vi "Lookup Manager.vi"(8 "error in (no error)":errorcluster, 11 "GUI Helper in":refnum<class "GUI Helper.lvclass">) -> (0 "error out":errorcluster, 3 "GUI Helper out":refnum<class "GUI Helper.lvclass">)   [LabVIEW 2020, in "VolatusGUI.lvlib" / "GUI Helper.lvclass"]
uses:
  GUI Helper.lvclass
  C:/dev/lv20CE/relink/lv-volatus/Volatus/Module/Module.lvclass
  Volatus/GUI Manager Identity/GUI Manager Identity.lvclass
  C:/dev/lv20CE/relink/lv-volatus/Volatus/Identity/Identity.lvclass
  Volatus/Module/Module.lvclass/Module.ctl
  GUI Helper.lvclass/GUI Helper.ctl
  GUI Registration.ctl
  Volatus/MessageQ/MessageQ.lvclass
  Volatus/MessageQ/MessageQ.lvclass/MessageQ.ctl
  Volatus/VolatusAPI/VolatusAPI.lvclass
  Volatus/Module/Module.lvclass
  VolatusGUI.lvlib
  GUI Info.ctl
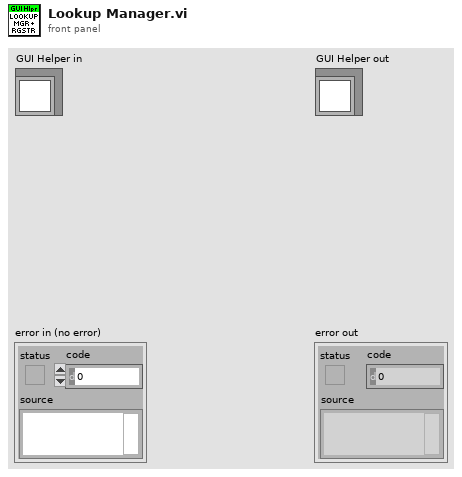
[diagram p1: front panel]
types:
  T1 = typedef "VolatusGUI.lvlib/GUI Info.ctl" = cluster{"Color":u32, "Name":string}
  T2 = typedef "VolatusGUI.lvlib/GUI Registration.ctl" = cluster{"ID":string, "GUI Helper":refnum<class "MessageQ.lvclass">, "Module":refnum<class "MessageQ.lvclass">, "Info":T1}
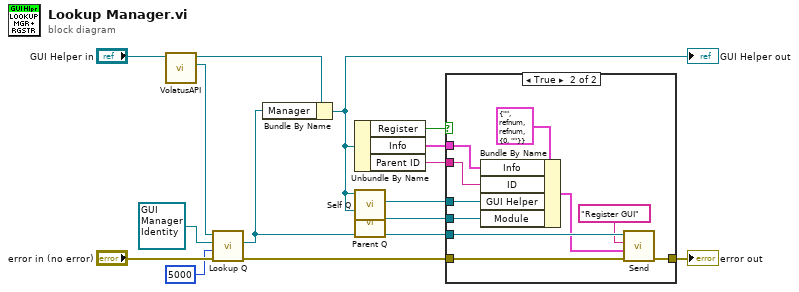
[diagram p0: block diagram]
diagram:
  n1 = call "VolatusAPI.vi"("Module in"="GUI Helper in") -> ("VolatusAPI"=w13:refnum<class "VolatusAPI.lvclass">, "Module out"=w11:refnum<class "GUI Helper.lvclass">)  [unwired: 9 in]
  n2 = call "Lookup Q.vi"("error in (no error)"="error in (no error)", "Timeout ms (0)"=5000, "Identity"=refnum<class "GUI Manager Identity.lvclass"> refnum ("VolatusGUI:GUI Manager Identity.lvclass"), "VolatusAPI in"=w13) -> ("error out"=w8:errorcluster, "MessageQ"=w7:refnum<class "MessageQ.lvclass">)  [unwired: 5 in, 1 out]
  n3 = Bundle By Name(cluster=w11, "Manager"=w7) -> (w9:refnum<class "GUI Helper.lvclass">)
  "GUI Helper out" <- w9
  n4 = Unbundle By Name(w9) -> ("Register"=w2:bool, "Info"=w1:T1, "Parent ID"=w3:string)
  n5 = call "Self Q.vi"("Module in"=w9) -> ("Self Q"=w5:refnum<class "MessageQ.lvclass">)  [unwired: 9 in, 1 out]
  n6 = call "Parent Q.vi"("Module in"=w9) -> ("Parent Q"=w4:refnum<class "MessageQ.lvclass">)  [unwired: 9 in, 1 out]
  n7 = case shown="True" w2 {
    tunnel: w8 -> [w16 w26]
    tunnel: w7 -> [_ w25]
    tunnel: [w16 w23] -> w6
    tunnel: w5 -> [_ w21]
    tunnel: w4 -> [_ w20]
    tunnel: w3 -> [_ w19]
    tunnel: w1 -> [_ w17]
    frame False {
    }
    frame True {
      n8 = Bundle By Name(cluster=T2 {"ID"="", "GUI Helper"=refnum, "Module"=refnum, "Info"={"Color"=0, "Name"=""}} ("GUI Registration"), "Info"=w17, "ID"=w19, "GUI Helper"=w21, "Module"=w20) -> (w18:T2)
      n9 = call "Send.vi"("error in (no error)"=w26, "Data"=w18, "ID"="Register GUI", "MessageQ in"=w25) -> ("error out"=w23:errorcluster)  [unwired: 6 in, 1 out]
    }
  }
  "error out" <- w6
